vi "clearScheduler.vi"() -> (0 "Empty Waveform":waveform(dbl), 1 "Empty Waveform Graphs":waveform(dbl)[](array[waveform]), 2 "Empty Scheduler":T1(array[cluster]))   [LabVIEW 2018]
panel:
  in  "Empty Scheduler Constant":T1(array[cluster])=[{"time (s)"=0.0, "setpoint "=0.0, "frequency"=0.0}]
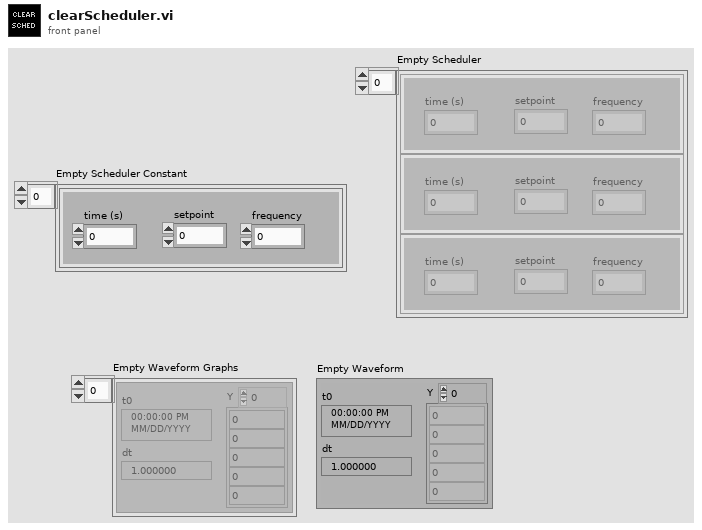
[diagram p1: front panel]
types:
  T1 = cluster{"time (s)":dbl, "setpoint ":dbl, "frequency":dbl}[]
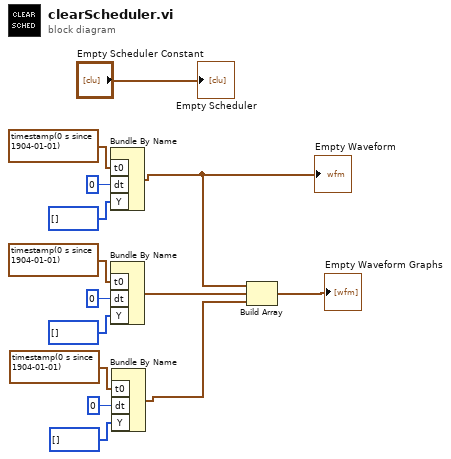
[diagram p0: block diagram]
diagram:
  n1 = Bundle By Name("t0"=timestamp(0 s since 1904-01-01), "dt"=0, "Y"=i32[] []) -> (w3:waveform(i32))  [unwired: 1 in]
  "Empty Waveform" <- w3
  n2 = Bundle By Name("t0"=timestamp(0 s since 1904-01-01), "dt"=0, "Y"=i32[] []) -> (w2:waveform(i32))  [unwired: 1 in]
  n3 = Bundle By Name("t0"=timestamp(0 s since 1904-01-01), "dt"=0, "Y"=i32[] []) -> (w1:waveform(i32))  [unwired: 1 in]
  n4 = Build Array(w3, w2, w1) -> (→"Empty Waveform Graphs":waveform(i32)[])
  "Empty Scheduler" <- "Empty Scheduler Constant"
